vi "Wait For Motion Done.vi"(8 "error in (no error)":errorcluster, 10 "Axis":i32=1, 11 "VISA resource name":refnum<visa-resource-name>) -> (0 "error out":errorcluster, 3 "VISA resource name out":refnum<visa-resource-name>)   [LabVIEW 2015]
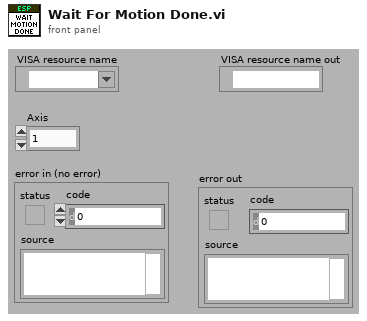
[diagram p1: front panel]
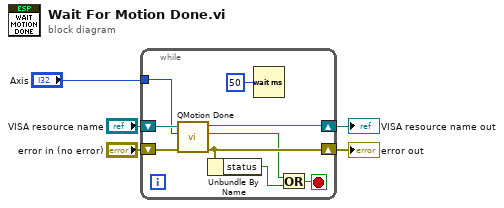
[diagram p0: block diagram]
diagram:
  n1 = while {
    shift-right: [w12] -> w1
    shift-left: "VISA resource name" -> [w14]
    shift-right: [w11] -> w2
    shift-left: "error in (no error)" -> [w13]
    tunnel: "Axis" -> [w6]
    stop <- w8 stop-if-true
    n2 = call "QMotion Done.vi"("error in (no error)"=w13, "Axis"=w6, "VISA resource name in"=w14) -> ("error out"=w11:errorcluster, "Motion Done?"=w9:bool, "VISA resource name out"=w12:refnum<visa-resource-name>)  [unwired: 6 in]
    n3 = Unbundle By Name(w11) -> ("status"=w10:bool)
    n4 = Wait (ms)(milliseconds to wait=u32 50) -> ()  [unwired: 1 out]
    n5 = Or(x=w9, y=w10) -> (x .or. y?=w8:bool)
  }
  "error out" <- w2
  "VISA resource name out" <- w1
